vi "Acquisition Started.vi"(8 "error in (no error)":errorcluster, 11 "HIJ Vision Camera App in":refnum<class "HIJ Vision Camera App.lvclass">) -> (0 "error out":errorcluster, 3 "HIJ Vision Camera App out":refnum<class "HIJ Vision Camera App.lvclass">)   [LabVIEW 2020, in "HIJ Vision Camera App.lvlib" / "HIJ Vision Camera App.lvclass"]
uses:
  HIJ Vision Camera App.lvclass
  HIJ Vision Camera App.lvclass/HIJ Vision Camera App.ctl
  <vilib>/ActorFramework/Message Enqueuer/Message Priority.ctl
  <vilib>/ActorFramework/Message Enqueuer/Message Enqueuer.lvclass
  Camera Actors/Camera Actor/ICamera Messages/Acquisition Started Msg/Acquisition Started Msg.lvclass
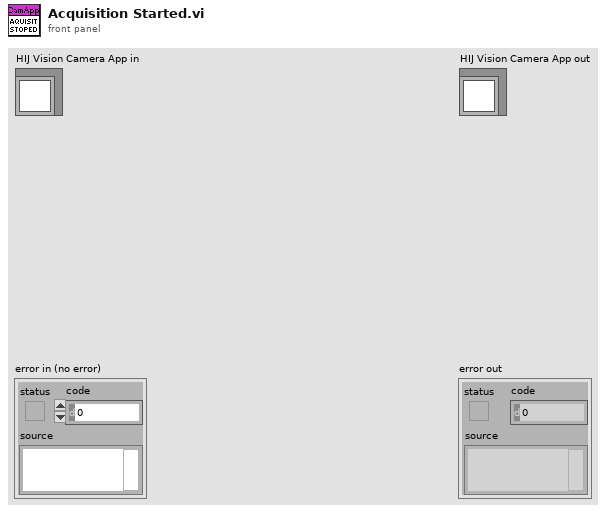
[diagram p1: front panel]
types:
  T1 = typedef "Actor Framework.lvlib/Message Enqueuer.lvclass/Message Priority.ctl" = enum16{"Low", "Normal", "High"}
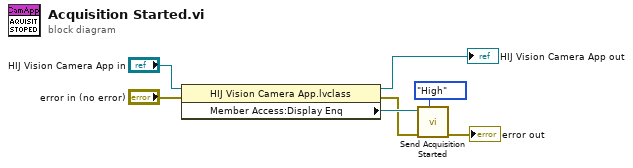
[diagram p0: block diagram]
diagram:
  n1 = property class="HIJ Vision Camera App.lvclass"(reference="HIJ Vision Camera App in", error in="error in (no error)") -> (reference out=→"HIJ Vision Camera App out":refnum<class "HIJ Vision Camera App.lvclass">, error out=w2:errorcluster, "Member Access:Display Enq"=w6:refnum<class "Message Enqueuer.lvclass">)
  n2 = call "Send Acquisition Started.vi"("Message Priority (Normal)"=Message_Priority."High", "error in (no error)"=w2, "Message Enqueuer"=w6) -> ("error out"=→"error out":errorcluster)  [unwired: 7 in, 1 out]
